vi "LM35_Thermostat_without_Hysteresis.vi"() -> ()   [LabVIEW 2019]
uses:
  <vilib>/Utility/error.llb/DialogType.ctl
  <vilib>/Instr/_visa.llb/VISA Configure Serial Port (Instr).vi
panel:
  out "RELAY STATUS":bool
  out "read buffer":string="\r\n"
  in  "STOP":bool
  in  "VISA resource name":refnum<visa-resource-name>="COM4"
  out "Waveform Chart":cluster{dbl, dbl}(graph)={26.3, 22.95}
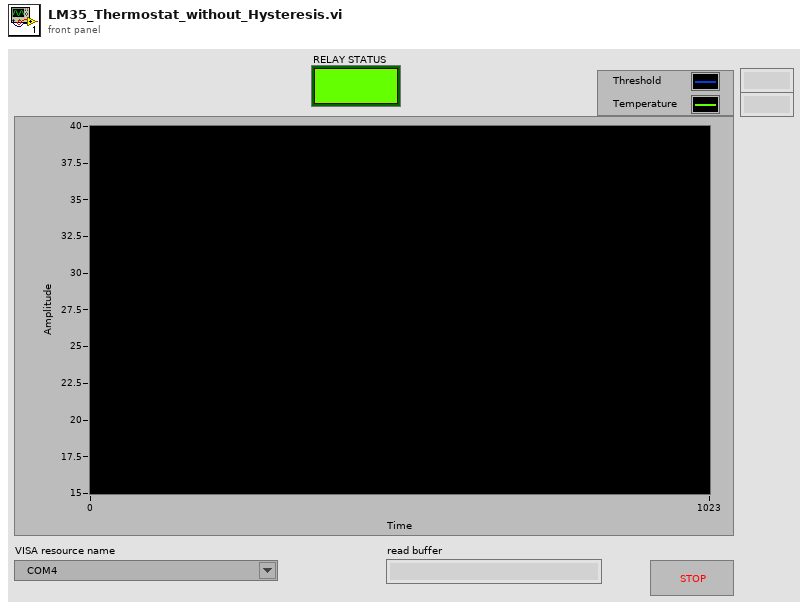
[diagram p1: front panel]
types:
  T1 = typedef "DialogType.ctl" = u16
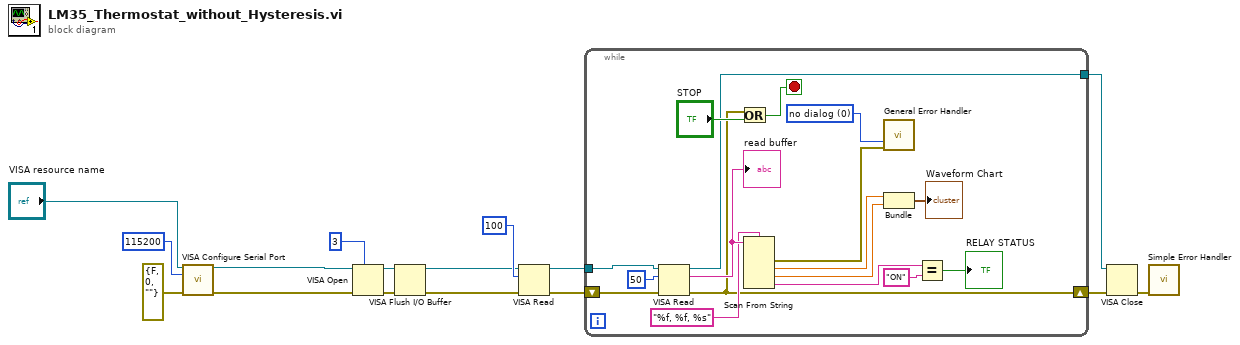
[diagram p0: block diagram]
diagram:
  n1 = call-poly "VISA Configure Serial Port"("VISA resource name"="VISA resource name", "baud rate (9600)"=u32 115200, "error in (no error)"=errorcluster {"status"=FALSE, "code"=0, "source"=""}) -> ("VISA resource name out"=w14:refnum<visa-resource-name>, "error out"=w15:errorcluster)  [unwired: 11 in]
  n2 = VISA Open(timeout (0)=u32 3 ("VISA Open timeout (0)"), error in (no error)=w15, VISA resource name=w14) -> (VISA resource name=w4:refnum<visa-resource-name>, error out=w3:errorcluster)  [unwired: 2 in]
  n3 = VISA Flush I/O Buffer(VISA resource name=w4, error in (no error)=w3) -> (VISA resource name out=w1:refnum<visa-resource-name>, error out=w2:errorcluster)  [unwired: 1 in]
  n4 = VISA Read(VISA resource name=w1, byte count=u32 100, error in (no error)=w2) -> (VISA resource name out=w8:refnum<visa-resource-name>, error out=w7:errorcluster)  [unwired: 2 out]
  n5 = while {
    tunnel: w8 -> [w33]
    tunnel: [w29] -> w11
    shift-right: [w23] -> w13
    shift-left: w7 -> [w32]
    stop <- w31 stop-if-true
    w21 = T1 0 items=["no dialog", "OK message", "continue or stop message", "OK message + warnings", "continue/stop + warnings"] ("type of dialog (OK msg:1)")
    n6 = VISA Read(VISA resource name=w33, byte count=u32 50, error in (no error)=w32) -> (VISA resource name out=w29:refnum<visa-resource-name>, read buffer=w28:string, error out=w23:errorcluster)  [unwired: 1 out]
    "read buffer" <- w28
    n7 = Or(x=w23, y="STOP") -> (x .or. y?=w31:bool)
    n8 = Scan From String "Scan From String"(format string="%f, %f, %s", input string=w28) -> (error out=w22:errorcluster, output 1=w26:dbl, output 2=w25:dbl, output 3=w19:string)  [unwired: 5 in, 2 out]
    n9 = call <vilib>:"General Error Handler.vi"("type of dialog (OK msg:1)"=w21, "error in (no error)"=w22) -> ()  [unwired: 9 in, 5 out]
    n10 = Bundle(w26, w25) -> (→"Waveform Chart":cluster{dbl, dbl})  [unwired: 1 in]
    n11 = Equal?(x=w19, y="ON") -> (x = y?=→"RELAY STATUS":bool)
  }
  n12 = VISA Close(VISA resource name=w11, error in (no error)=w13) -> (error out=w12:errorcluster)
  n13 = call <vilib>:"Simple Error Handler.vi"("error in (no error)"=w12) -> ()  [unwired: 4 in, 5 out]
